vi "Custom Control Folder.vi"(9 "operation":enum16{"Get", "Set"}(ring), 11 "custom control folder":path) -> (3 "custom control folder out":path)   [LabVIEW 2018, in "NISAST VI Scripting.lvlib" / "VI.lvlib" / "Front Panel.lvlib"]
uses:
  Front Panel.lvlib
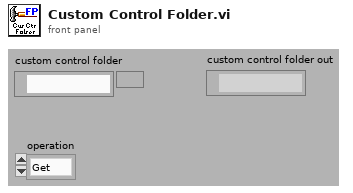
[diagram p1: front panel]
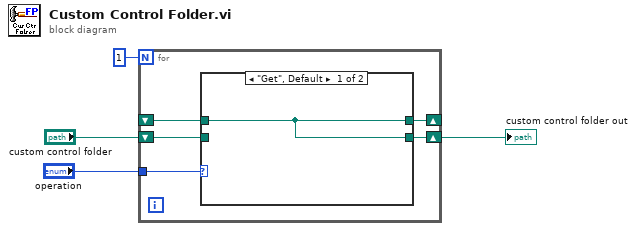
[diagram p0: block diagram]
diagram:
  n1 = for {
    N: 1 -> [_]
    shift-right: [w8] -> _
    shift-left: _ -> [w7]
    tunnel: "operation" -> [w9]
    shift-right: [w5] -> w2
    shift-left: "custom control folder" -> [w6]
    n2 = case shown="\"Get\", Default" w9 {
      tunnel: [w10 w11] -> w8
      tunnel: w7 -> [w10 _]
      tunnel: w6 -> [_ w11]
      tunnel: [w10 w11] -> w5
      frame "Get", Default {
      }
      frame "Set" {
      }
    }
  }
  "custom control folder out" <- w2
